vi "Search_file_content.vi"() -> ()   [LabVIEW 2011]
panel:
  out "Matched string":string
  in  "offset (0)":i32
  out "offset past match":i32
  in  "Filename":path
  out "after substring":string
  out "before substring":string
  in  "regular expression":string
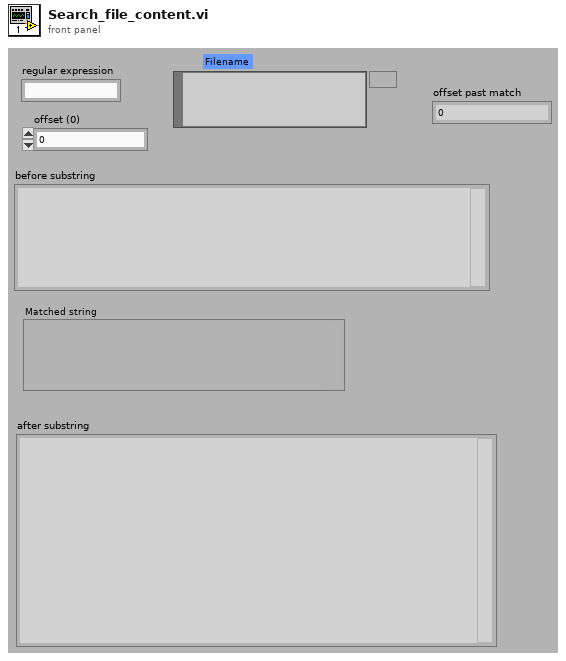
[diagram p1: front panel]
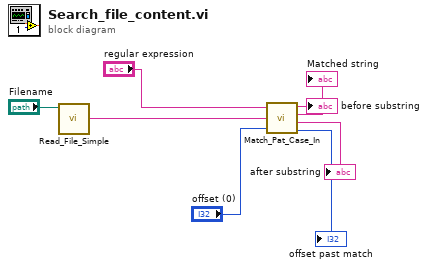
[diagram p0: block diagram]
diagram:
  n1 = call "Read_File_Simple.vi"("Filename"="Filename") -> ("string"=w3:string)  [unwired: 4 in, 5 out]
  n2 = call "Match_Pat_Case_In.vi"("String to match"="regular expression", "String"=w3, "offset (0)"="offset (0)") -> ("Before Matched string"=→"before substring":string, "Matched string"=→"Matched string":string, "After  Matched string"=→"after substring":string, "offset past match"=→"offset past match":i32)
